vi "4.6.4.vi"() -> ()   [LabVIEW 2017]
panel:
  in  "停止":bool
  out "数值 3":dbl
  in  "数值 2":dbl
  in  "数值":dbl
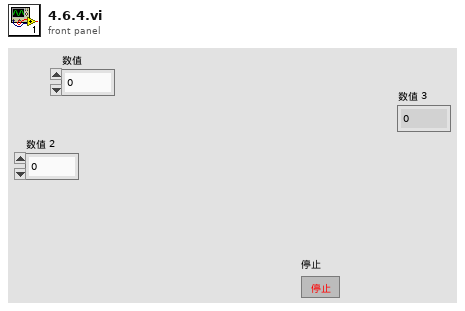
[diagram p1: front panel]
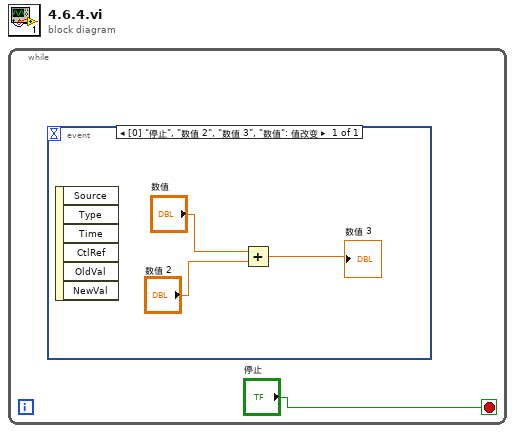
[diagram p0: block diagram]
diagram:
  n1 = while {
    stop <- "停止" stop-if-true
    n2 = event shown="[0] \"停止\", \"数值 2\", \"数值 3\", \"数值\": 值改变" {
      selector: _ -> [_]
      dyn-events: _ -> [_]
      timeout: _ -> [_]
      event "停止", "数值 2", "数值 3", "数值": Value Change {
        n3 = event-data() -> ()  [unwired: 1 in, 6 out]
        n4 = Add(x="数值", y="数值 2") -> (x+y=→"数值 3":dbl)
      }
    }
  }
